vi "3_32_Fxp_addation.vi"(1 "y":fxp<+/-,32,3>, 2 "x":fxp<+/-,32,3>) -> (0 "x+y":fxp<+/-,33,4> format="%.41g")   [LabVIEW 2020]
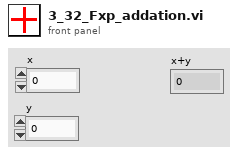
[diagram p1: front panel]
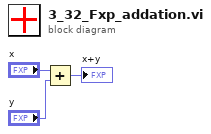
[diagram p0: block diagram]
diagram:
  n1 = Add(x="x", y="y") -> (x+y=→"x+y":fxp<+/-,33,4>)
